vi "DriveToTarget.vi"(8 "error in (no error)":errorcluster) -> (0 "error out":errorcluster)   [LabVIEW 2016]
uses:
  Robot Global Data.vi
  Drive Base Class/DriveBase.lvclass
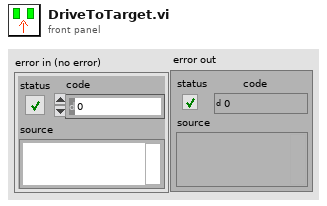
[diagram p1: front panel]
types:
  T1 = cluster{"Lower X":dbl, "Lower Y":dbl, "Upper X":dbl, "Upper Y":dbl, "Lower Limit":dbl, "Upper Limit":dbl}
  T2 = cluster{"Target?":bool, "PegAngle":dbl, "Distance":dbl}
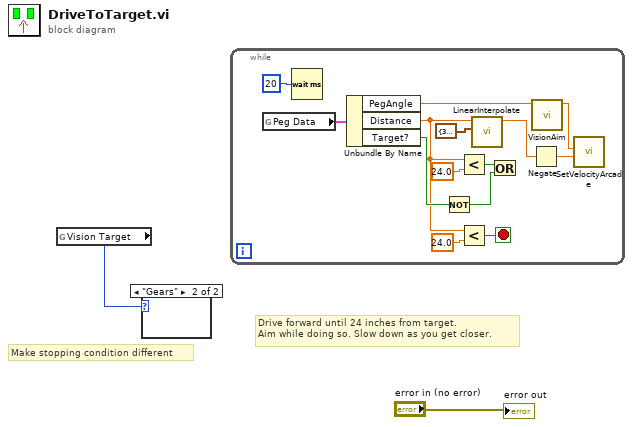
[diagram p0: block diagram]
diagram:
  # "Make stopping condition different"
  # "Drive forward until 24 inches from target.\nAim while doing so. Slow down as you get closer."
  n1 = global read "Robot Global Data.vi" "Vision Target"() -> (w2:enum16{"Pegs", "Gears"})
  n2 = case shown="\"Gears\"" w2 {
    frame "Pegs", Default {
    }
    frame "Gears" {
    }
  }
  n3 = while {
    stop <- w6 stop-if-true
    n4 = global read "Robot Global Data.vi" "Peg Data"() -> (w14:T2)
    n5 = Wait (ms)(milliseconds to wait=u32 20) -> ()  [unwired: 1 out]
    n6 = Unbundle By Name(w14) -> ("PegAngle"=w13:dbl, "Distance"=w5:dbl, "Target?"=w10:bool)
    n7 = Not(x=w10) -> (.not. x?=w11:bool)
    n8 = Less?(x=w5, y=24.0) -> (x < y?=w12:bool)
    n9 = Less?(x=w5, y=24.0) -> (x < y?=w6:bool)
    n10 = call "LinearInterpolate.vi"("Config"=T1 {"Lower X"=30.0, "Lower Y"=0.4, "Upper X"=60.0, "Upper Y"=0.75, "Lower Limit"=0.4, "Upper Limit"=0.75}, "Value"=w5) -> ("Ouput"=w8:dbl)  [unwired: 9 in]
    n11 = Or(x=w12, y=w11) -> ()  [unwired: 1 out]
    n12 = Negate(x=w8) -> (-x=w4:dbl)
    n13 = call "VisionAim.vi"("Angle"=w13) -> ("Turn Amount"=w3:dbl)  [unwired: 9 in, 1 out]
    n14 = call "SetVelocityArcade.vi"("Y Axis"=w4, "X Axis"=w3) -> ()  [unwired: 9 in, 1 out]
  }
  "error out" <- "error in (no error)"
